vi "FTW-ActorExtended-Connection-Ask.vi"(0 "FTW-ActorExtended In":refnum<class "FTW-ActorExtended.lvclass">, 5 "Connector Name":string, 7 "Message Header":string, 9 "Message Body":string, 11 "error in":errorcluster, 12 "Timeout":i32=1000 format="%dmsec") -> (4 "FTW-ActorExtended Out":refnum<class "FTW-ActorExtended.lvclass">, 6 "Response Header":string, 8 "Response Body":string, 10 "Timed out?":bool, 14 "Roundtrip Time":dbl format="%.6fsec", 15 "error out":errorcluster)   [LabVIEW 2013, in "FTW-ActorExtended.lvclass"]
uses:
  FTW-ActorExtended.lvclass
  FTW-ActorExtended.lvclass/FTW-ActorExtended.ctl
  Connector/FTW-ActorConnector.lvclass
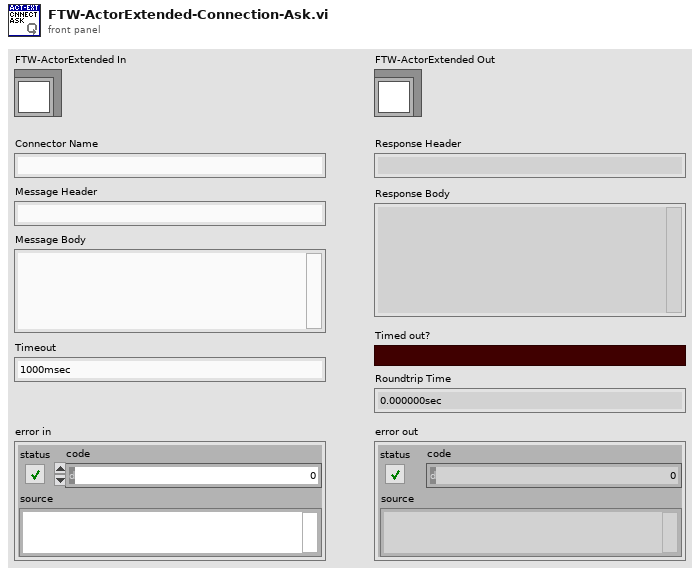
[diagram p1: front panel]
types:
  T1 = cluster{"Name":string, "URI":string, "Connector":refnum<class "FTW-ActorConnector.lvclass">}[]
  T2 = cluster{"Name":string, "URI":string, "Connector":refnum<class "FTW-ActorConnector.lvclass">}
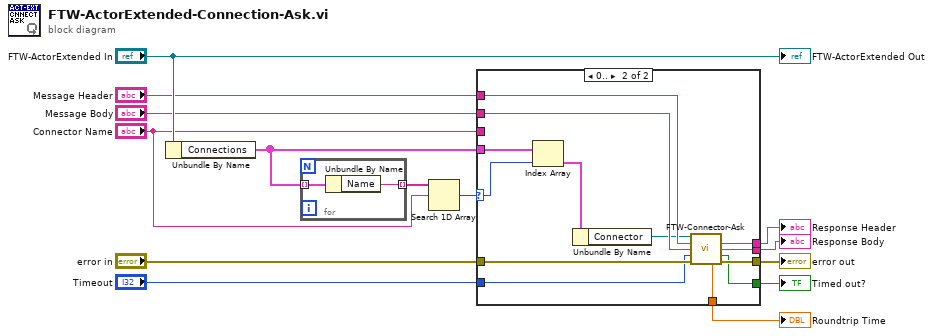
[diagram p0: block diagram]
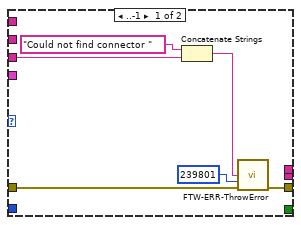
[diagram p2: hidden frame]
diagram:
  n1 = Unbundle By Name("FTW-ActorExtended In") -> ("Connections"=w12:T1)
  n2 = for {
    tunnel: w12 -> [w16] mode=indexing
    tunnel: [w15] -> w2 mode=indexing
    n3 = Unbundle By Name(w16) -> ("Name"=w15:string)
  }
  n4 = Search 1D Array(1D array=w2, element="Connector Name") -> (index of element=w13:i32)  [unwired: 1 in]
  n5 = case shown="0.." w13 {
    selector: w13 -> [_ w35]
    tunnel: w12 -> [_ w34]
    tunnel: [w21 w32] -> w11
    tunnel: "error in" -> [w22 w33]
    tunnel: "Connector Name" -> [w17 _]
    tunnel: "Message Header" -> [_ w31]
    tunnel: "Message Body" -> [_ w30]
    tunnel: [_ w29] -> w6
    tunnel: [_ w28] -> w5
    tunnel: [_ w27] -> w4
    tunnel: [_ w26] -> w3
    tunnel: "Timeout" -> [_ w23]
    frame ..-1 {
      n6 = Concatenate Strings("Could not find connector " ("Error Message"), w17) -> (w18:string)
      n7 = call "FTW-ERR-ThrowError.vi"("Error Message"=w18, "Error Code"=239801, "error in"=w22) -> ("error out"=w21:errorcluster)  [unwired: 12 in]
    }
    frame 0.. {
      n8 = Index Array(array=w34, index=w35) -> (element=w25:T2)
      n9 = Unbundle By Name(w25) -> ("Connector"=w24:refnum<class "FTW-ActorConnector.lvclass">)
      n10 = call "FTW-Connector-Ask.vi"("FTW Actor Connector"=w24, "Request Header"=w31, "Request Body"=w30, "Timeout"=w23, "error in"=w33) -> ("Response Header"=w26:string, "Response Body"=w27:string, "Timed out?"=w28:bool, "Roundtrip Time"=w29:dbl, "error out"=w32:errorcluster)  [unwired: 5 in, 1 out]
    }
  }
  "error out" <- w11
  "Timed out?" <- w5
  "Response Header" <- w3
  "Response Body" <- w4
  "Roundtrip Time" <- w6
  "FTW-ActorExtended Out" <- "FTW-ActorExtended In"
